vi "_Read ADC.vi"(1 "Channel #":i8) -> ()   [LabVIEW 2015]
uses:
  Type/_FPGA Chip Type.ctl
  <vilib>/rvi/eio/common/nirviEmuTemplateMethod_errors.vi
  <vilib>/rvi/Memory/Memory_Emulation/nirvimemoryEmulation.vi
  <vilib>/rvi/Memory/Memory_Emulation/nirvimemoryFastEmulation.vi
  <vilib>/rvi/DataTransferAndStorage/Container/Common/niFpgaContainerGetUniqueNameForEmu.vi
  <vilib>/rvi/Memory/Memory_Emulation/niFpgaMemoryEmulationCacheClearOnFirstRun.vi
  <vilib>/rvi/Memory/Memory_Emulation/nirvimemoryEmulationManagerCache_MakeExclusive.vi
  <vilib>/rvi/Memory/Memory_Emulation/niFpgaMemoryEmulationValidateCache.vi
  <vilib>/rvi/Memory/Memory_Emulation/nirvimemoryEmulationManagerCache_InsertValue.vi
  <vilib>/Utility/error.llb/Clear Errors.vi
  <vilib>/rvi/Memory/Memory_Emulation/nirvimemoryEmulationManagerCache_ReleaseExclusive.vi
  <vilib>/rvi/Memory/Memory_Emulation/nirvimemoryEmulationManagerCache_GetValue.vi
  <vilib>/rvi/Emulation/niFpgaEmulationIsFPGAContextNoSignature.vi
  <vilib>/rvi/Emulation/niFpgaSctlEmulationGetInTimedLoop.vi
  <vilib>/rvi/Memory/Memory_Emulation/nirvimemoryEmulationManagerCache_SetValue.vi
  <vilib>/rvi/Emulation/niFpgaSctlEmulationResourceMgr.vi
  <vilib>/rvi/Emulation/niFpgaGetClockAttributes.vi
  <vilib>/rvi/Emulation/niFpgaEmulationReportErrorSimple.vi
  <vilib>/rvi/Emulation/niFpgaCriticalErrorInLSC.vi
  <vilib>/eio/EIONode/EIONode.xnode
  <vilib>/rvi/DataTransferAndStorage/Container/XNode/niFpgaContainer.xnode
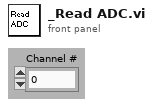
[diagram p1: front panel]
types:
  T1 = typedef "_FPGA Chip Type.ctl" = enum8{"None", "ADC1", "ADC2", "ADC3", "ADC4", "ADC5", "ADC6", "ADC7", "ADC8", "ADC9", "ADC10", "ADC11", "ADC12", "ADC13", "DAC1", "DAC2", "DAC3", "DAC4", "DAC5", "LENS1", "LENS2", "LENS3", "LENS4", "LENS5", "LENS6", "LENS7", "MASS1", "MASS2", "MASS3", "MASS4", "MASS5", "OSC1", "OSC2", "OSC3", "LATCH1", "LATCH2", "LATCH3", "LATCH4", "PIC1", "PIC2", "PIC3", "PIC4"}
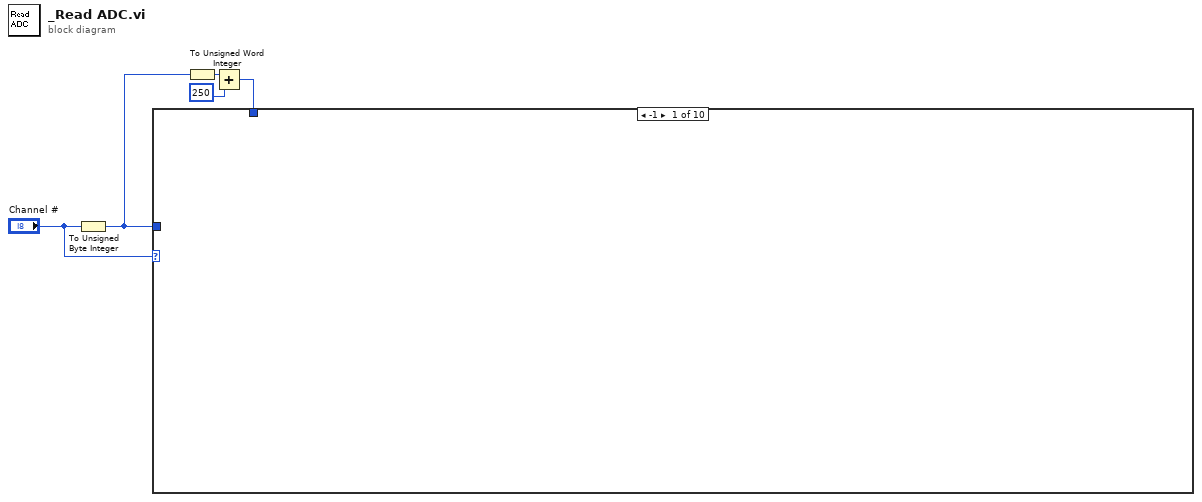
[diagram p0: block diagram]
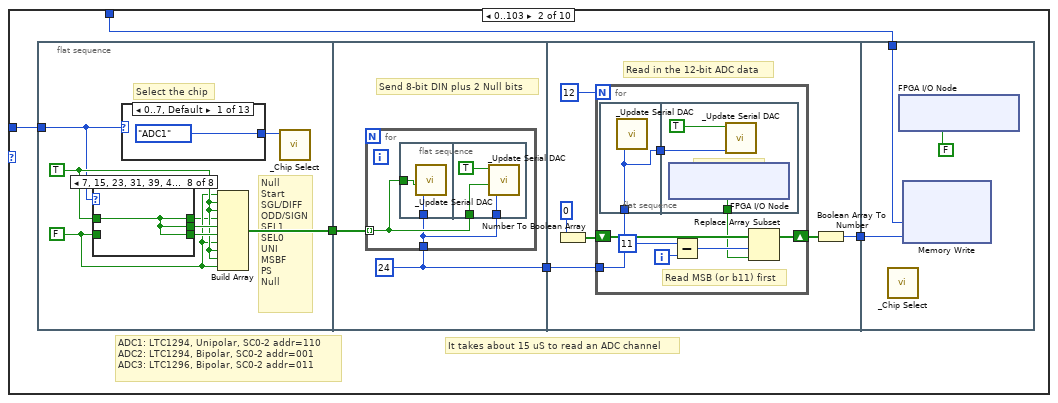
[diagram p2: hidden frame]
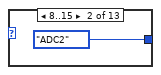
[diagram p10: hidden frame]
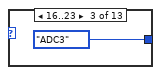
[diagram p11: hidden frame]
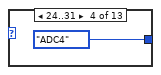
[diagram p12: hidden frame]
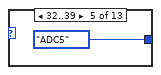
[diagram p13: hidden frame]
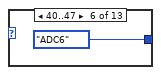
[diagram p14: hidden frame]
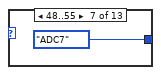
[diagram p15: hidden frame]
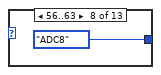
[diagram p16: hidden frame]
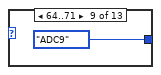
[diagram p17: hidden frame]
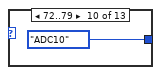
[diagram p18: hidden frame]
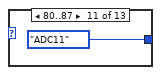
[diagram p19: hidden frame]
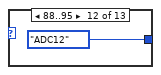
[diagram p20: hidden frame]
diagram:
  n1 = To Unsigned Byte Integer(number="Channel #") -> (unsigned 8bit integer=w2:u8)
  n2 = To Unsigned Word Integer(number=w2) -> (unsigned 16bit integer=w5:u16)
  n3 = Add(x=w5, y=u16 250 ("Timeout (-1 for no timeout)")) -> (x+y=w3:u16)
  n4 = case shown="-1" "Channel #" {
    tunnel: w2 -> [_ w8 w81 w84 _ _ _ _ _ _]
    tunnel: w3 -> [_ w7 w80 _ _ w94 w97 w100 w103 w106]
    frame -1 {
    }
    frame 0..103 {
      # "It takes about 15 uS to read an ADC channel"
      # "ADC1: LTC1294, Unipolar, SC0-2 addr=110\nADC2: LTC1294, Bipolar, SC0-2 addr=001\nADC3: LTC1296, Bipolar, SC0-2 addr=011"
      n5 = flat-sequence {
        tunnel: [w16] -> w10
        tunnel: w8 -> [w11]
        tunnel: w10 -> [w47]
        tunnel: [w46] -> w6
        tunnel: [w56] -> w9
        tunnel: w6 -> [w55]
        tunnel: w9 -> [w75]
        tunnel: w7 -> [w74]
        frame #0 {
          w13 = FALSE
          w15 = TRUE
          # "Null\nStart\nSGL/DIFF\nODD/SIGN\nSEL1\nSEL0\nUNI\nMSBF\nPS\nNull"
          # "Select the chip"
          n6 = case shown="7, 15, 23, 31, 39, 47, 55, 63, 71, 79, 87, 95, 103" w11 {
            tunnel: [w19 w21 w23 w25 w26 w29 w30 w32] -> w12
            tunnel: [w19 w20 w23 w24 w27 w29 w31 w32] -> w18
            tunnel: [w19 w20 w22 w25 w26 w28 w31 w32] -> w17
            tunnel: w15 -> [_ w21 w22 w25 w27 w29 w31 w32]
            tunnel: w13 -> [w19 w20 w23 w24 w26 w28 w30 _]
            frame 0, 8, 16, 24, 32, 40, 48, 56, 64, 72, 80, 88, 96, Default {
            }
            frame 1, 9, 17, 25, 33, 41, 49, 57, 65, 73, 81, 89, 97 {
            }
            frame 2, 10, 18, 26, 34, 42, 50, 58, 66, 74, 82, 90, 98 {
            }
            frame 3, 11, 19, 27, 35, 43, 51, 59, 67, 75, 83, 91, 99 {
            }
            frame 4, 12, 20, 28, 36, 44, 52, 60, 68, 76, 84, 92, 100 {
            }
            frame 5, 13, 21, 29, 37, 45, 53, 61, 69, 77, 85, 93, 101 {
            }
            frame 6, 14, 22, 30, 38, 46, 54, 62, 70, 78, 86, 94, 102 {
            }
            frame 7, 15, 23, 31, 39, 47, 55, 63, 71, 79, 87, 95, 103 {
            }
          }
          n7 = case shown="0..7, Default" w11 {
            tunnel: [_FPGA_Chip_Type."ADC1" ("ChipType") _FPGA_Chip_Type."ADC2" ("ChipType") _FPGA_Chip_Type."ADC3" ("ChipType") _FPGA_Chip_Type."ADC4" ("ChipType") _FPGA_Chip_Type."ADC5" ("ChipType") _FPGA_Chip_Type."ADC6" ("ChipType") _FPGA_Chip_Type."ADC7" ("ChipType") _FPGA_Chip_Type."ADC8" ("ChipType") _FPGA_Chip_Type."ADC9" ("ChipType") _FPGA_Chip_Type."ADC10" ("ChipType") _FPGA_Chip_Type."ADC11" ("ChipType") _FPGA_Chip_Type."ADC12" ("ChipType") _FPGA_Chip_Type."ADC13" ("ChipType")] -> w14
            frame 0..7, Default {
            }
            frame 8..15 {
            }
            frame 16..23 {
            }
            frame 24..31 {
            }
            frame 32..39 {
            }
            frame 40..47 {
            }
            frame 48..55 {
            }
            frame 56..63 {
            }
            frame 64..71 {
            }
            frame 72..79 {
            }
            frame 80..87 {
            }
            frame 88..95 {
            }
            frame 96..103 {
            }
          }
          n8 = Build Array(w13, w15, w15, w12, w18, w17, w13, w15, w15, w13) -> (w16:bool[])
          n9 = call "_Chip Select.vi"("ChipType"=w14) -> ()  [unwired: 1 in, 6 out]
        }
        frame #1 {
          w46 = u8 24 ("Wait(12Ticks)")
          # "Send 8-bit DIN plus 2 Null bits"
          n10 = for {
            tunnel: w47 -> [w49] mode=indexing
            tunnel: w46 -> [w48]
            n11 = flat-sequence {
              tunnel: w49 -> [w51]
              tunnel: w48 -> [w50]
              tunnel: w49 -> [w54]
              tunnel: w48 -> [w52]
              frame #0 {
                n12 = call "_Update Serial DAC.vi"("Wait(12Ticks)"=w50, "DIN (F)"=w51) -> ()  [unwired: 2 in, 4 out]
              }
              frame #1 {
                n13 = call "_Update Serial DAC.vi"("Wait(12Ticks)"=w52, "DIN (F)"=w54, "Clock (F)"=TRUE ("Clock")) -> ()  [unwired: 1 in, 4 out]
              }
            }
          }
        }
        frame #2 {
          # "Read in the 12-bit ADC data"
          n14 = Number To Boolean Array(number=u16 0) -> (Boolean array=w58:bool[])
          n15 = for {
            N: 12 -> [_]
            shift-right: [w67] -> w57
            shift-left: w58 -> [w68]
            tunnel: w55 -> [w62]
            i -> [w66]
            # "Read MSB (or b11) first"
            n16 = flat-sequence {
              tunnel: w62 -> [w69]
              tunnel: [w69] -> w61
              tunnel: [w71] -> w63
              tunnel: w61 -> [w70]
              frame #0 {
                n17 = call "_Update Serial DAC.vi"("Wait(12Ticks)"=w69) -> ()  [unwired: 3 in, 4 out]
              }
              frame #1 {
                # "Read SDOUT"
                n18 = xnode "FPGA I/O Node"() -> ("Digtal IO/DIO7"=w71:bool)  [unwired: 1 in, 1 out]
                n19 = call "_Update Serial DAC.vi"("Wait(12Ticks)"=w70, "Clock (F)"=TRUE ("Clock")) -> ()  [unwired: 2 in, 4 out]
              }
            }
            n20 = Subtract(x=11, y=w66) -> (x-y=w64:i32)
            n21 = Replace Array Subset(array=w68, new element=w63, index=w64) -> (w67:bool[])
          }
          n22 = Boolean Array To Number(Boolean array=w57) -> (number=w56:u16)
        }
        frame #3 {
          n23 = call "_Chip Select.vi"() -> ()  [unwired: 2 in, 6 out]
          n24 = xnode "FPGA I/O Node"("Digtal IO/DIO9"=FALSE ("Port1/DIO0")) -> ()  [unwired: 1 in, 1 out]
          n25 = xnode ("Memory Write")("Address"=w74, "Data"=w75) -> ()  [unwired: 1 in, 1 out]
        }
      }
    }
    frame 104..110 {
      # "Read PIC channels"
      n26 = xnode ("Memory Read")("Address"=w80) -> ("Data"=w77:u32)  [unwired: 1 in, 1 out]
      n27 = Split Number(x=w77) -> (hi(x)=w76:u16)  [unwired: 1 out]
      n28 = Subtract(x=w81, y=u8 24) -> (x-y=w78:u8)
      n29 = call "_Set 1 DAC Value.vi"("DAC"=w76, "Ch#"=w78) -> ()  [unwired: 2 out]
    }
    frame 113, 114 {
      # "Read Source ID"
      n30 = Subtract(x=w84, y=u8 24) -> (x-y=w82:u8)
      n31 = while {
        tunnel: w82 -> [w92]
        i -> [w86]
        stop <- w89 stop-if-true
        w85 = u8 2 ("upper limit")
        n32 = call "_Set 1 DAC Value.vi"("Ch#"=w92) -> ("PIC Monitor"=w91:u8)  [unwired: 1 in, 1 out]
        n33 = Greater Or Equal?(x=w86, y=w85) -> (x >= y?=w87:bool)
        n34 = In Range and Coerce(upper limit=w85, x=w91, lower limit=u8 0) -> (In Range?=w88:bool)  [unwired: 1 out]
        n35 = Or(x=w88, y=w87) -> (x .or. y?=w89:bool)
      }
    }
    frame 115, Default {
      # "No need to read the -ve PIC channels\nas they are the same as the +ve channels"
    }
    frame 119 {
      # "Read VAC Gauge"
      n36 = call "_Read VAC Gauge.vi"() -> ("DAC"=w93:u8)
      n37 = xnode ("Memory Write")("Address"=w94, "Data"=w93) -> ()  [unwired: 1 in, 1 out]
    }
    frame 120 {
      # "Read Card Cage Door Interlock"
      n38 = xnode "FPGA I/O Node"() -> ("Digtal IO/DIO60"=w96:bool)  [unwired: 1 in, 1 out]
      n39 = Boolean To (0,1)(Boolean=w96) -> (0, 1=w95:i16)
      n40 = xnode ("Memory Write")("Address"=w97, "Data"=w95) -> ()  [unwired: 1 in, 1 out]
    }
    frame 121 {
      # "Read Vacuum Ready"
      n41 = xnode "FPGA I/O Node"() -> ("Digtal IO/DIO6"=w99:bool)  [unwired: 1 in, 1 out]
      n42 = Boolean To (0,1)(Boolean=w99) -> (0, 1=w98:i16)
      n43 = xnode ("Memory Write")("Address"=w100, "Data"=w98) -> ()  [unwired: 1 in, 1 out]
    }
    frame 126 {
      # "LC1 In"
      n44 = xnode "FPGA I/O Node"() -> ("Digtal IO/DIO51"=w102:bool)  [unwired: 1 in, 1 out]
      n45 = Boolean To (0,1)(Boolean=w102) -> (0, 1=w101:i16)
      n46 = xnode ("Memory Write")("Address"=w103, "Data"=w101) -> ()  [unwired: 1 in, 1 out]
    }
    frame 127 {
      # "LC2 In"
      n47 = xnode "FPGA I/O Node"() -> ("Digtal IO/DIO53"=w105:bool)  [unwired: 1 in, 1 out]
      n48 = Boolean To (0,1)(Boolean=w105) -> (0, 1=w104:i16)
      n49 = xnode ("Memory Write")("Address"=w106, "Data"=w104) -> ()  [unwired: 1 in, 1 out]
    }
  }
